vi "Connect.vi"(8 "error in (no error)":errorcluster, 10 "Channel(s)":string, 11 "Hioki9002 Switch":refnum<class "Hioki9002.lvclass">) -> (0 "error out":errorcluster, 3 "Hioki9002 Switch":refnum<class "Hioki9002.lvclass">)   [LabVIEW 2019, in "Concrete.lvlib" / "Hioki9002.lvclass"]
uses:
  Hioki9002.lvclass
  Hioki9002.lvclass/Hioki9002.ctl
  Harware Abstraction/Switch/Switch.lvclass
  <instrlib>/HIOKI SW100X Series/HIOKI SW100X Series.lvlib
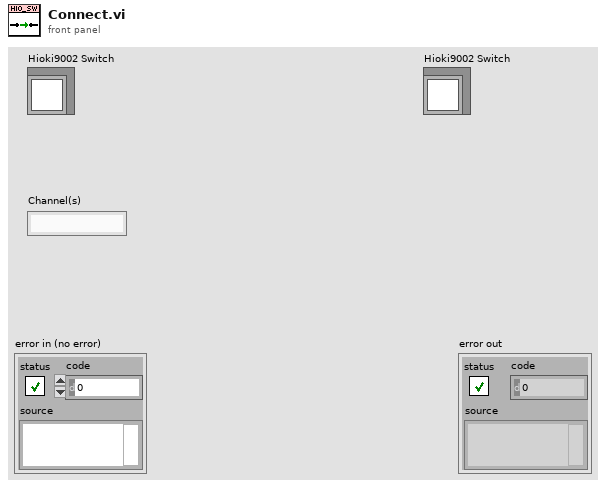
[diagram p1: front panel]
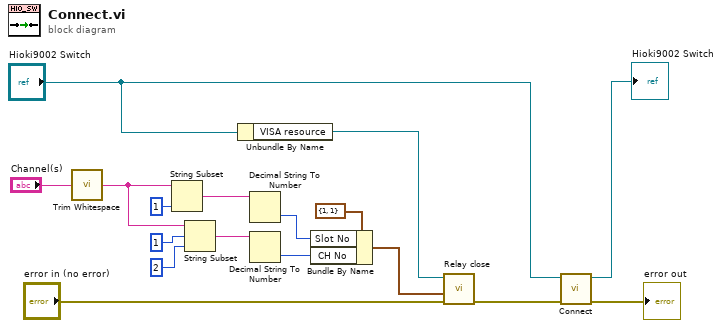
[diagram p0: block diagram]
diagram:
  n1 = call <vilib>:"Trim Whitespace.vi"("string"="Channel(s)") -> ("trimmed string"=w5:string)  [unwired: 1 in]
  n2 = String Subset(string=w5, length (rest)=1 ("length (rest)")) -> (substring=w6:string)  [unwired: 1 in]
  n3 = String Subset(string=w5, offset (0)=1, length (rest)=2 ("length (rest)")) -> (substring=w3:string)
  n4 = Unbundle By Name("Hioki9002 Switch") -> ("VISA resource"=w14:refnum<visa-resource-name>)
  n5 = Decimal String To Number(string=w6) -> (number=w10:i32)  [unwired: 2 in, 1 out]
  n6 = Decimal String To Number(string=w3) -> (number=w9:i32)  [unwired: 2 in, 1 out]
  n7 = Bundle By Name(cluster=cluster{"Slot No":u16, "CH No":u16} {"Slot No"=1, "CH No"=1} ("Close Point"), "Slot No"=w10, "CH No"=w9) -> (w12:cluster{"Slot No":u16, "CH No":u16})
  n8 = call <instrlib>:"Relay close.vi"("error in"="error in (no error)", "Close Point"=w12, "VISA resource name"=w14) -> ("error out"=w15:errorcluster)  [unwired: 6 in, 2 out]
  n9 = call-parent "Connect.vi"("error in (no error)"=w15, "Switch in"="Hioki9002 Switch") -> ("error out"=→"error out":errorcluster, "Switch out"=→"Hioki9002 Switch":refnum<class "Hioki9002.lvclass">)  [unwired: 8 in]
